vi "Up-Left Vector Check.vi"(8 "Column":i32, 9 "Row":i32, 10 "Opponent's Tiles":bool[][](array[boolean]), 11 "Current Player's Tiles":bool[][](array[boolean])) -> (2 "Possible Flips":T1[](array[typedef]), 3 "Possible Location":bool)   [LabVIEW 2020, in "Reversi.lvlib" / "Reversi.lvclass"]
uses:
  Reversi.lvclass
  Space Coordinates.ctl
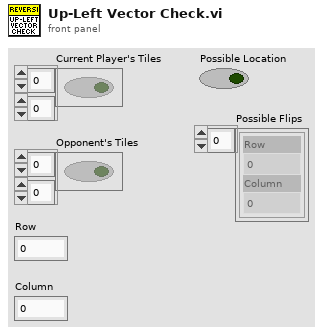
[diagram p1: front panel]
types:
  T1 = typedef "Reversi.lvlib/Reversi.lvclass/Space Coordinates.ctl" = cluster{"Row":i32, "Column":i32}
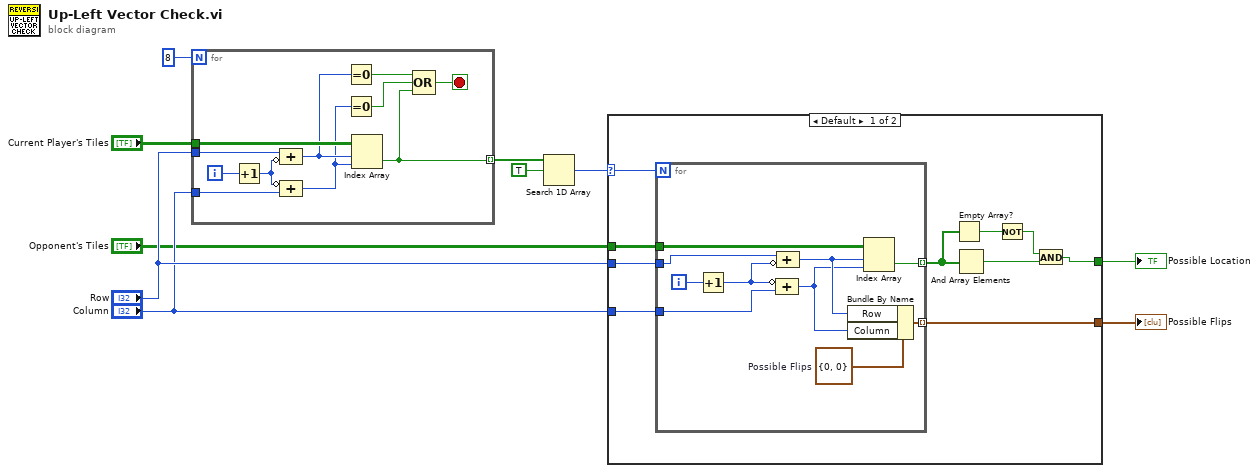
[diagram p0: block diagram]
diagram:
  n1 = for {
    N: 8 -> [_]
    tunnel: [w17] -> w9 mode=indexing
    tunnel: "Current Player's Tiles" -> [w21]
    tunnel: "Column" -> [w12]
    tunnel: "Row" -> [w19]
    i -> [w20]
    stop <- w16 stop-if-true
    n2 = Increment(x=w20) -> (x+1=w13:i32)
    n3 = Compound Arithmetic op=ADD(w19, invert w13) -> (w14:i32)
    n4 = Compound Arithmetic op=ADD(invert w13, w12) -> (w11:i32)
    n5 = Equal To 0?(x=w14) -> (x = 0?=w18:bool)
    n6 = Equal To 0?(x=w11) -> (x = 0?=w15:bool)
    n7 = Index Array(array=w21, index (row)=w14, index (col)=w11) -> (element=w17:bool)
    n8 = Compound Arithmetic op=OR(w18, w15, w17) -> (w16:bool)
  }
  n9 = Search 1D Array(1D array=w9, element=TRUE) -> (index of element=w2:i32)  [unwired: 1 in]
  n10 = case shown="Default" w2 {
    selector: w2 -> [w22 _]
    tunnel: "Opponent's Tiles" -> [w27 _]
    tunnel: "Column" -> [w25 _]
    tunnel: [w28 _] -> w6
    tunnel: "Row" -> [w26 _]
    tunnel: [w23 _] -> w10
    frame Default {
      n11 = for {
        N: w22 -> [_]
        tunnel: [w39] -> w24 mode=indexing
        tunnel: w27 -> [w41]
        tunnel: w26 -> [w38]
        tunnel: w25 -> [w32]
        tunnel: [w37] -> w23 mode=indexing
        i -> [w40]
        w35 = T1 {"Row"=0, "Column"=0}  # Possible Flips
        n12 = Increment(x=w40) -> (x+1=w34:i32)
        n13 = Compound Arithmetic op=ADD(invert w34, w32) -> (w33:i32)
        n14 = Compound Arithmetic op=ADD(w38, invert w34) -> (w36:i32)
        n15 = Bundle By Name(cluster=w35, "Row"=w36, "Column"=w33) -> (w37:T1)
        n16 = Index Array(array=w41, index (row)=w36, index (col)=w33) -> (element=w39:bool)
      }
      n17 = Empty Array?(array=w24) -> (empty?=w31:bool)
      n18 = And Array Elements(Boolean array=w24) -> (logical AND=w29:bool)
      n19 = Not(x=w31) -> (.not. x?=w30:bool)
      n20 = And(x=w30, y=w29) -> (x .and. y?=w28:bool)
    }
    frame -1 {
    }
  }
  "Possible Flips" <- w10
  "Possible Location" <- w6
